vi "Master__Main.vi"() -> ()   [LabVIEW 2018]
doc: "Main VI to be run from cRIO controller. Must be started after the HostMain.vi on host computer.\n\nFirst function starts the bitfile on the FPGA which operates a watchdog.\nFollowed by Master_Initializer which puts all of the outputs and variables into a safe state, to prevent any unintended actuations or executions. If there are any faults in the initalization, the vi will skip to Master_Shutdown, which sets all variables to a safe state and aborts the bitfile.\nIf the initialization is successful, four parallel loops are operated: Control, DAQ, IMU, CAN.\n\nThe control loop reads commands from Host__Main.vi and also operates the main state machine for semi-autonomously controlling the pod. It also contains fault checking and pets/kicks the watchdog.\nThe DAQ loop reads analog input data from the c-series module and compiles that into the data cluster. It combines that cluster with clusters containing IMU, BMS, and motor controller data before setting it into a network shared variable to be read by the host.\nThe IMUMain loop reads and parses strings sent by the IMU via RS232 to the cRIO's serial port.\nThe CAN loop contains CAN-related subvis to establish a connection, and parse data from the BMS and motor controller."
uses:
  <vilib>/Utility/error.llb/DialogType.ctl
  <vilib>/FPGAPlugInAG/cRIO-9063/niLvFpga_Open_cRIO-9063.vi
  <vilib>/rvi/interface/common/dynamic/niFpgaDynamicAddResources.vi
  <vilib>/FPGAPlugInAG/Dynamic/niLvFpga_Run_Dynamic.vi
  <vilib>/FPGAPlugInAG/Dynamic/niLvFpga_Abort_Dynamic.vi
  <vilib>/FPGAPlugInAG/Dynamic/niLvFpga_Close_Dynamic.vi
  <vilib>/rvi/interface/nirviOpenFPGA/nirviOpenFPGA.xnode
  FPGA Bitfiles/TheMacroProject_FPGATarget_Fail-SafeControl_eeRwxioMFzY.lvbitx
  <vilib>/rvi/interface/nirviMethod/nirviMethod.xnode
  <vilib>/rvi/interface/nirviCloseFPGA/nirviCloseFPGA.xnode
panel:
  out "error out":errorcluster
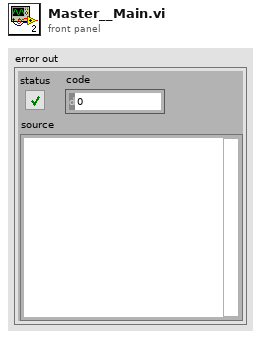
[diagram p1: front panel]
types:
  T1 = typedef "DialogType.ctl" = u16
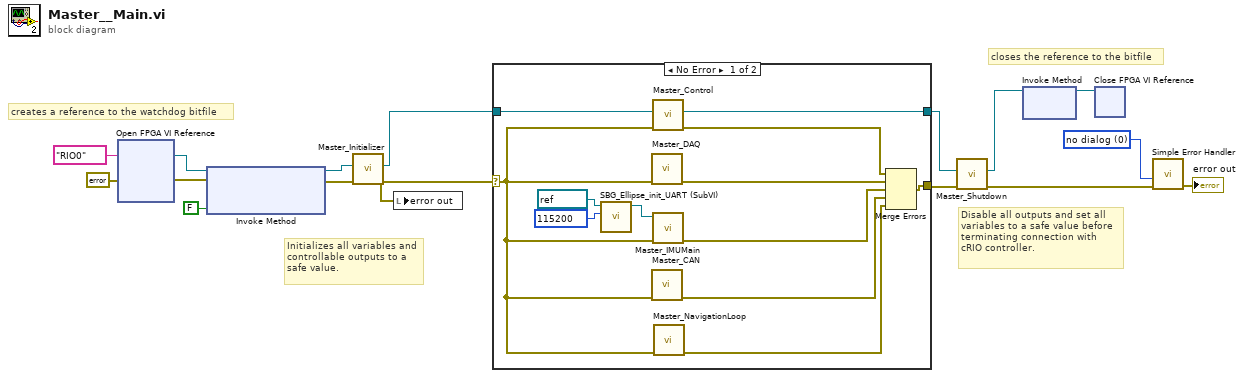
[diagram p0: block diagram]
diagram:
  w16 = T1 0 items=["no dialog", "OK message", "continue or stop message", "OK message + warnings", "continue/stop + warnings"] ("type of dialog (OK msg:1)")
  # "closes the reference to the bitfile"
  # "creates a reference to the watchdog bitfile"
  # "Disable all outputs and set all\nvariables to a safe value before\nterminating connection with \ncRIO controller."
  # "Initializes all variables and\ncontrollable outputs to a \nsafe value."
  n1 = xnode "Open FPGA VI Reference"("error in"=errorcluster {"status"=FALSE, "code"=0, "source"=""}, "resource name"=tag "RIO0") -> ("FPGA VI Reference Out"=w8:refnum<k20>, "error out"=w13:errorcluster)
  n2 = xnode "Invoke Method"("FPGA VI Reference In"=w8, "error in"=w13, "Wait Until Done (F)"=FALSE) -> ("FPGA VI Reference Out"=w1:refnum<k20>, "error out"=w12:errorcluster)
  n3 = call "Master_Initializer.vi"("error in (no error)"=w12, "FPGA VI Reference In"=w1) -> ("error out"=w5:errorcluster, "FPGA VI Reference Out"=w7:refnum<k20>)  [unwired: 8 in]
  n4 = local write "error out"(w5) -> ()
  n5 = case shown="No Error" w5 {
    selector: w5 -> [w17 w30]
    tunnel: [w23 w30] -> w15
    tunnel: [w24 w29] -> w4
    tunnel: w7 -> [w25 w29]
    frame No Error {
      w28 = u32 115200 items=["9600"=9600, "19200"=19200, "36400"=36400, "57600"=57600, "115200"=115200, "230400"=230400, "460800"=460800, "921600"=921600] ("Baudrate")
      n6 = call "SBG_Ellipse_init_UART (SubVI).vi"("Baudrate"=w28, "VISA Refnum in"=refnum<visa-resource-name> "IMU" ("VISA resource name")) -> ("VISA Refnum out"=w26:refnum<visa-resource-name>)  [unwired: 8 in, 1 out]
      n7 = call "Master_DAQ.vi"("error in (no error)"=w17) -> ("error out"=w21:errorcluster)  [unwired: 10 in]
      n8 = call "Master_CAN.vi"("error in"=w17) -> ("error out"=w18:errorcluster)  [unwired: 10 in]
      n9 = call "Master_Control.vi"("error in (no error)"=w17, "FPGA VI Reference In"=w25) -> ("error out"=w20:errorcluster, "FPGA VI Reference Out"=w24:refnum<k20>)  [unwired: 8 in]
      n10 = call "Master_IMUMain.vi"("error in"=w17, "VISA Refnum out"=w26) -> ("error out"=w22:errorcluster)  [unwired: 9 in]
      n11 = call "Master_NavigationLoop.vi"("error in (no error)"=w17) -> ("error out"=w19:errorcluster)  [unwired: 10 in]
      n12 = Merge Errors(w20, w21, w22, w18, w19) -> (w23:errorcluster)
    }
    frame Error {
    }
  }
  n13 = call "Master_Shutdown.vi"("error in"=w15, "FPGA VI Reference In"=w4) -> ("error out"=w2:errorcluster, "FPGA VI Reference Out"=w3:refnum<k20>)  [unwired: 8 in]
  n14 = xnode "Invoke Method"("FPGA VI Reference In"=w3) -> ("FPGA VI Reference Out"=w10:refnum<k20>)  [unwired: 1 in, 1 out]
  n15 = xnode "Close FPGA VI Reference"("FPGA VI Reference In"=w10) -> ()  [unwired: 1 in, 1 out]
  n16 = call <vilib>:"Simple Error Handler.vi"("type of dialog (OK msg:1)"=w16, "error in (no error)"=w2) -> ("error out"=→"error out":errorcluster)  [unwired: 3 in, 4 out]
